vi "photo_encoder_laggy.vi"() -> ()   [LabVIEW 2014]
panel:
  out "Marks/second":i16
  in  "Brightness of Mark":dbl
  in  "Photo Value(placeholder for sensor data)":dbl
  # "This VI recognizes significant increases in brightness as \"marks\" and outputs the number of marks detected in the last second.\nUpdates one second late."
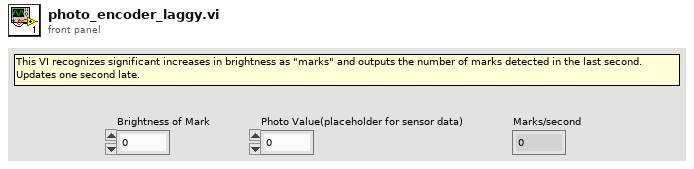
[diagram p1: front panel]
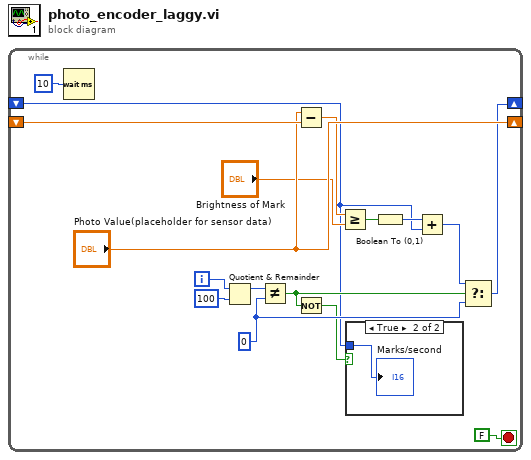
[diagram p0: block diagram]
diagram:
  n1 = while {
    shift-right: ["Photo Value(placeholder for sensor data)"] -> _
    shift-left: _ -> [w17]
    shift-right: [w4] -> _
    shift-left: _ -> [w1]
    i -> [w8]
    stop <- FALSE stop-if-true
    w5 = i16 0 ("f")
    n2 = Wait (ms)(milliseconds to wait=u32 10) -> ()  [unwired: 1 out]
    n3 = Quotient & Remainder(x=w8, y=100) -> (x-y*floor(x/y)=w6:i32)  [unwired: 1 out]
    n4 = Not Equal?(x=w6, y=w5) -> (x != y?=w2:bool)
    n5 = Subtract(x="Photo Value(placeholder for sensor data)", y=w17) -> (x-y=w15:dbl)
    n6 = Not(x=w2) -> (.not. x?=w3:bool)
    n7 = Greater Or Equal?(x=w15, y="Brightness of Mark") -> (x >= y?=w11:bool)
    n8 = case shown="True" w3 {
      tunnel: w1 -> [_ w18]
      frame False {
      }
      frame True {
        "Marks/second" <- w18
      }
    }
    n9 = Boolean To (0,1)(Boolean=w11) -> (0, 1=w10:i16)
    n10 = Add(x=w10, y=w1) -> (x+y=w9:i16)
    n11 = Select(t=w9, s=w2, f=w5) -> (s? t:f=w4:i16)
  }
